vi "KE622x -- Get Triax Inner Shield Connection.vi"(0 "Resource In":refnum<visa-resource-name>, 1 "Check For SCPI Errors? (T)":bool=TRUE, 11 "error in (no error)":errorcluster) -> (4 "Resource Out (dupl)":refnum<visa-resource-name>, 8 "Triax Inner Shield Connection":T1=enum."Cable Guard", 15 "error out":errorcluster)   [LabVIEW 2009, in "Keithley 622x.lvlib"]
doc: "Returns the connection point of the triax inner shield, either 'Output Low' or 'Cable Guard'. See the corresponding 'set' VI for a more detailed explanation of the inner shield connection."
uses:
  <instrlib>/Keithley 622x LV 2009/Keithley 622x.lvlib
  <instrlib>/Keithley 622x LV 2009/Configure/Output/Typedefs/KE622x -- Triax Inner Shield Connection.ctl
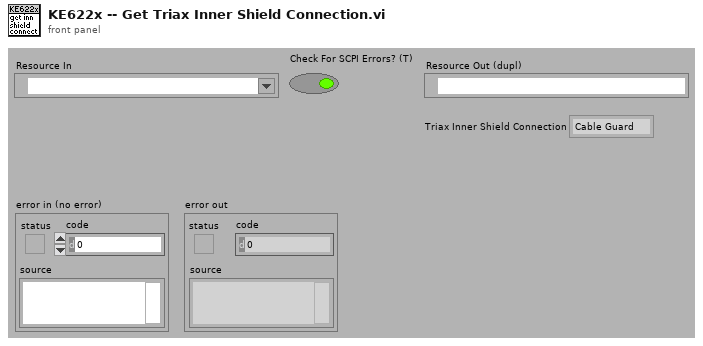
[diagram p1: front panel]
types:
  T1 = typedef "Keithley 622x.lvlib/KE622x -- Triax Inner Shield Connection.ctl" = enum16{"Output Low", "Cable Guard"}
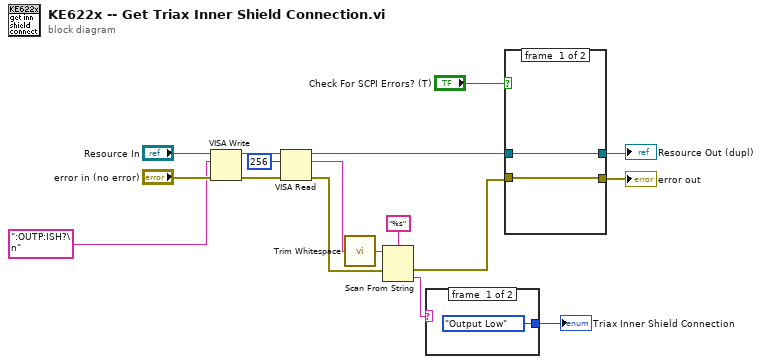
[diagram p0: block diagram]
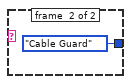
[diagram p2: hidden frame]
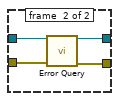
[diagram p3: hidden frame]
diagram:
  n1 = VISA Write(VISA resource name="Resource In", write buffer=":OUTP:ISH?\n" ("format string"), error in (no error)="error in (no error)") -> (VISA resource name out=w11:refnum<visa-resource-name>, error out=w10:errorcluster)  [unwired: 1 out]
  n2 = VISA Read(VISA resource name=w11, byte count=u32 256, error in (no error)=w10) -> (VISA resource name out=w4:refnum<visa-resource-name>, read buffer=w6:string, error out=w8:errorcluster)  [unwired: 1 out]
  n3 = call <vilib>:"Trim Whitespace.vi"("string"=w6) -> ("trimmed string"=w3:string)  [unwired: 1 in]
  n4 = Scan From String(format string="%s", input string=w3, error in=w8) -> (error out=w5:errorcluster, output 1=w2:string)  [unwired: 2 in, 2 out]
  n5 = case shown="\"OLOW\", Default" w2 {
    tunnel: [KE622x_--_Triax_Inner_Shield_Connection."Output Low" ("Triax Inner Shield Connection") KE622x_--_Triax_Inner_Shield_Connection."Cable Guard" ("Triax Inner Shield Connection")] -> w1
    frame #0 {
    }
    frame #1 {
    }
  }
  "Triax Inner Shield Connection" <- w1
  n6 = case shown="False" "Check For SCPI Errors? (T)" {
    tunnel: w4 -> [w21 w25]
    tunnel: w5 -> [w20 w24]
    tunnel: [w20 w23] -> w13
    tunnel: [w21 w22] -> w14
    frame #0 {
    }
    frame #1 {
      n7 = call <instrlib>:"Error Query.vi"("VISA Resource In"=w25, "error in (no error)"=w24) -> ("VISA Resource Out (dupl)"=w22:refnum<visa-resource-name>, "error out"=w23:errorcluster)  [unwired: 10 in, 2 out]
    }
  }
  "Resource Out (dupl)" <- w14
  "error out" <- w13
